vi "calibrate trap data V3RG.vi"(0 "array of calibration clusters":T4(array[cluster]) {"offset_y (mV)" format="%#_2g"; "kappa_y (pN/nm)" min=0.0 step=0.001 format="%#_2g"; "alpha_y (nm/V)" step=10.0 format="%#_3g"; "kappa_x (pN/nm)" min=0.0 step=0.001 format="%#_2g"; "offset_x (mV)" format="%#_2g"; "alpha_x (nm/V)" step=10.0 format="%#_3g"}, 3 "Trap position array":dbl[](array[numeric]), 4 "MCL offset scanning range (V)":T2={"Min X"=5.0, "Max X"=10.0, "Min Y"=5.0, "Max Y"=10.0, "Scan increment"=5.0}, 5 "Multi-MCL offset array":T1(array[cluster]), 6 "two trap offset values":T3={"Trap 1X offset"=array[501 elements], "Trap 2X offset"=array[501 elements]}, 7 "Dynamic offset update":bool, 8 "Multiple-MCL offset?":bool, 9 "x (true) or y (false)":bool, 10 "Data array":waveform(dbl)[](array[waveform]), 11 "Offset File step size":dbl) -> (1 "Positions out":dbl[][](array[numeric]), 2 "Forces out (pN)":dbl[][](array[numeric]))   [LabVIEW 2014]
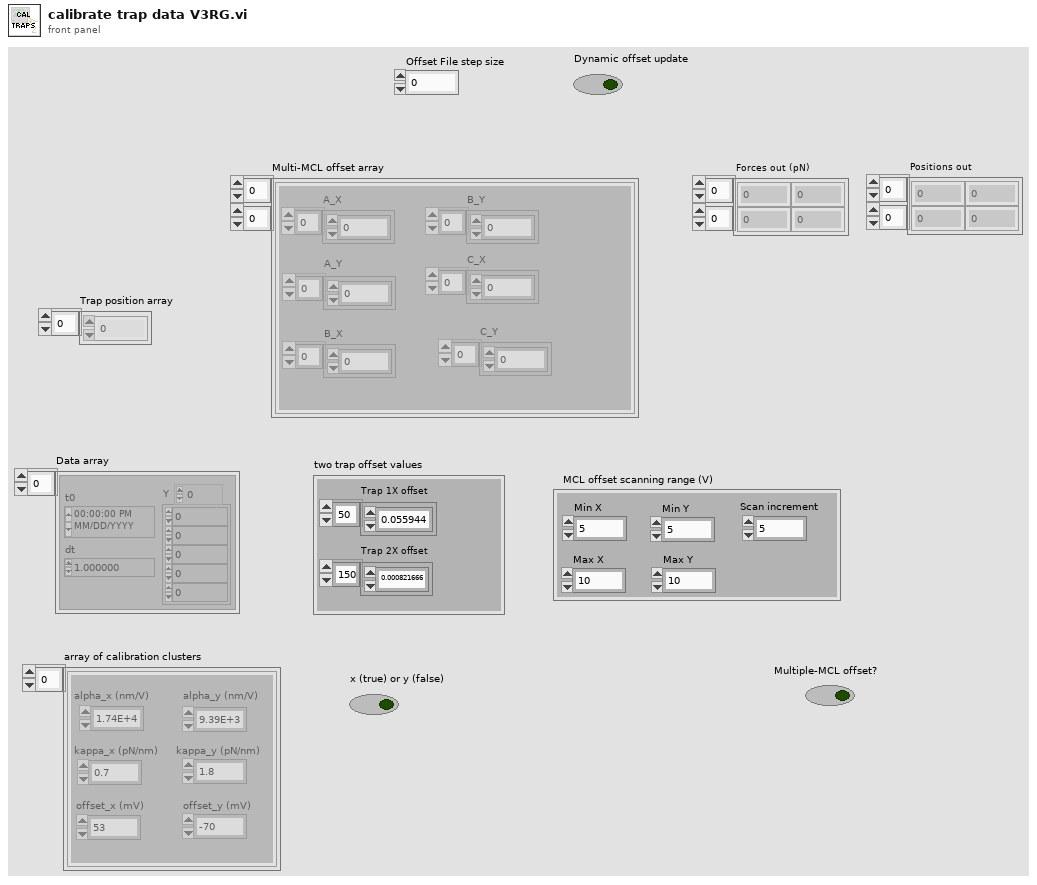
[diagram p1: front panel]
types:
  T1 = cluster{"A_X":dbl[], "A_Y":dbl[], "B_X":dbl[], "B_Y":dbl[], "C_X":dbl[], "C_Y":dbl[]}[][]
  T2 = cluster{"Min X":dbl, "Max X":dbl, "Min Y":dbl, "Max Y":dbl, "Scan increment":dbl}
  T3 = cluster{"Trap 1X offset":dbl[], "Trap 2X offset":dbl[]}
  T4 = cluster{"alpha_x (nm/V)":dbl, "offset_x (mV)":dbl, "kappa_x (pN/nm)":dbl, "alpha_y (nm/V)":dbl, "kappa_y (pN/nm)":dbl, "offset_y (mV)":dbl}[]
  T5 = cluster{"alpha_x (nm/V)":dbl, "offset_x (mV)":dbl, "kappa_x (pN/nm)":dbl, "alpha_y (nm/V)":dbl, "kappa_y (pN/nm)":dbl, "offset_y (mV)":dbl}
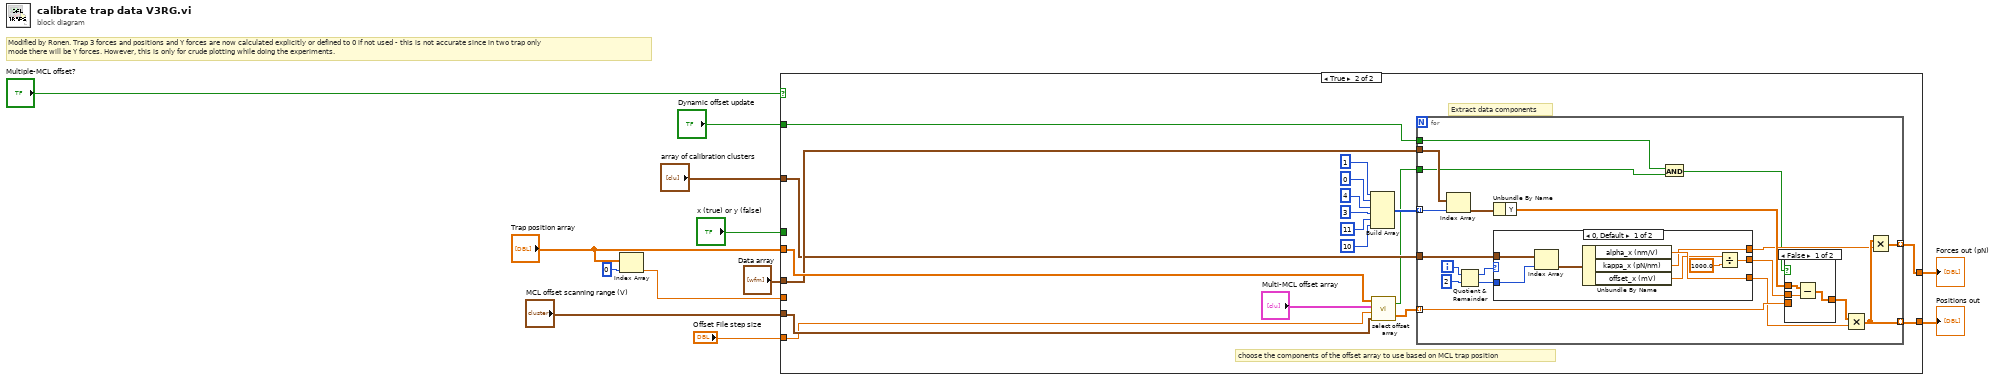
[diagram p0: block diagram]
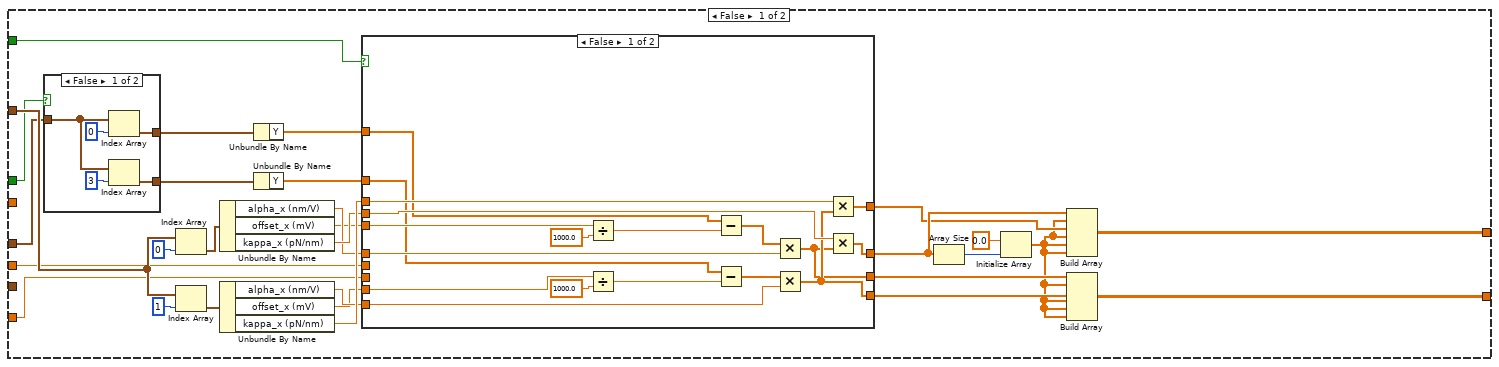
[diagram p2: hidden frame]
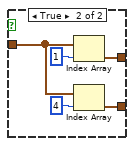
[diagram p3: hidden frame]
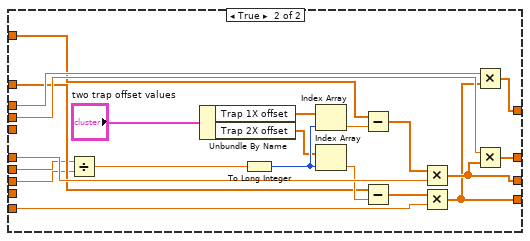
[diagram p4: hidden frame]
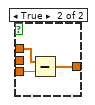
[diagram p5: hidden frame]
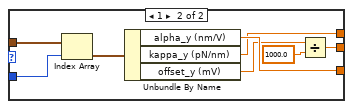
[diagram p6: hidden frame]
diagram:
  # "Modified by Ronen. Trap 3 forces and positions and Y forces are now calculated explicitly or defined to 0 if not used - this is not accurate since in two trap only\nmode there will be Y forces. However, this is only for crude plotting while doing the experiments."
  n1 = Index Array(array="Trap position array", index=0) -> (element=w7:dbl)
  n2 = case shown="True" "Multiple-MCL offset?" {
    tunnel: "Dynamic offset update" -> [w35 w94]
    tunnel: "array of calibration clusters" -> [w34 w95]
    tunnel: "Data array" -> [w29 w98]
    tunnel: w7 -> [w20 _]
    tunnel: "MCL offset scanning range (V)" -> [_ w107]
    tunnel: "Trap position array" -> [_ w108]
    tunnel: "Offset File step size" -> [w19 w97]
    tunnel: [w18 w92] -> w3
    tunnel: [w17 w93] -> w2
    tunnel: "x (true) or y (false)" -> [w16 _]
    frame False {
      n3 = case shown="False" w16 {
        tunnel: w29 -> [w43 w51]
        tunnel: [w44 w48] -> w28
        tunnel: [w42 w47] -> w27
        frame False {
          n4 = Index Array(array=w43, index=0) -> (element=w44:waveform(dbl))
          n5 = Index Array(array=w43, index=3) -> (element=w42:waveform(dbl))
        }
        frame True {
          n6 = Index Array(array=w51, index=1) -> (element=w48:waveform(dbl))
          n7 = Index Array(array=w51, index=4) -> (element=w47:waveform(dbl))
        }
      }
      n8 = Index Array(array=w34, index=0) -> (element=w31:T5)
      n9 = Index Array(array=w34, index=1) -> (element=w30:T5)
      n10 = Unbundle By Name(w31) -> ("alpha_x (nm/V)"=w38:dbl, "offset_x (mV)"=w36:dbl, "kappa_x (pN/nm)"=w40:dbl)
      n11 = Unbundle By Name(w30) -> ("alpha_x (nm/V)"=w39:dbl, "offset_x (mV)"=w37:dbl, "kappa_x (pN/nm)"=w41:dbl)
      n12 = Unbundle By Name(w28) -> ("Y"=w26:dbl[])
      n13 = Unbundle By Name(w27) -> ("Y"=w25:dbl[])
      n14 = case shown="False" w35 {
        tunnel: w36 -> [w63 _]
        tunnel: w37 -> [w62 _]
        tunnel: w38 -> [w61 w83]
        tunnel: w39 -> [w60 w80]
        tunnel: w40 -> [w59 w82]
        tunnel: w41 -> [w58 w79]
        tunnel: w25 -> [w57 w78]
        tunnel: w26 -> [w56 w77]
        tunnel: [w55 w73] -> w14
        tunnel: [w54 w74] -> w15
        tunnel: [w53 w75] -> w21
        tunnel: [w52 w76] -> w22
        tunnel: w20 -> [_ w71]
        tunnel: w19 -> [_ w70]
        frame False {
          n15 = Divide(x=w63, y=1000.0) -> (x/y=w67:dbl)
          n16 = Divide(x=w62, y=1000.0) -> (x/y=w66:dbl)
          n17 = Subtract(x=w56, y=w67) -> (x-y=w65:dbl[])
          n18 = Subtract(x=w57, y=w66) -> (x-y=w64:dbl[])
          n19 = Multiply(x=w65, y=w61) -> (x*y=w53:dbl[])
          n20 = Multiply(x=w64, y=w60) -> (x*y=w55:dbl[])
          n21 = Multiply(x=w58, y=w55) -> (x*y=w54:dbl[])
          n22 = Multiply(x=w59, y=w53) -> (x*y=w52:dbl[])
        }
        frame True {
          n23 = Divide(x=w71, y=w70) -> (x/y=w88:dbl)
          n24 = Unbundle By Name("two trap offset values") -> ("Trap 1X offset"=w85:dbl[], "Trap 2X offset"=w86:dbl[])
          n25 = To Long Integer(number=w88) -> (32bit integer=w87:i32)
          n26 = Index Array(array=w85, index=w87) -> (element=w84:dbl)
          n27 = Index Array(array=w86, index=w87) -> (element=w81:dbl)
          n28 = Subtract(x=w77, y=w84) -> (x-y=w90:dbl[])
          n29 = Subtract(x=w78, y=w81) -> (x-y=w89:dbl[])
          n30 = Multiply(x=w90, y=w83) -> (x*y=w75:dbl[])
          n31 = Multiply(x=w89, y=w80) -> (x*y=w73:dbl[])
          n32 = Multiply(x=w79, y=w73) -> (x*y=w74:dbl[])
          n33 = Multiply(x=w82, y=w75) -> (x*y=w76:dbl[])
        }
      }
      n34 = Array Size(array=w22) -> (size(s)=w24:i32)
      n35 = Initialize Array(0.0, w24) -> (w13:dbl[])
      n36 = Build Array(w22, w13, w15, w13, w13, w13) -> (w18:dbl[][])
      n37 = Build Array(w21, w13, w14, w13, w13, w13) -> (w17:dbl[][])
    }
    frame True {
      # "Extract data components"
      # "choose the components of the offset array to use based on MCL trap position"
      n38 = Build Array(1, 0, 4, 3, 11, 10) -> (w99:i32[])
      n39 = call "select offset array.vi"("MCL offset scanning range (V)"=w107, "Offset File step size"=w97, "Multi-MCL offset array"="Multi-MCL offset array", "Trap position array"=w108) -> ("Out offsets"=w96:dbl[], "In range?"=w91:bool)
      n40 = for {
        tunnel: w99 -> [w127] mode=indexing
        tunnel: w98 -> [w126]
        tunnel: w96 -> [w118] mode=indexing
        tunnel: w95 -> [w120]
        tunnel: w94 -> [w111]
        tunnel: [w114] -> w93 mode=indexing
        tunnel: [w112] -> w92 mode=indexing
        tunnel: w91 -> [w109]
        i -> [w123]
        n41 = Index Array(array=w126, index=w127) -> (element=w125:waveform(dbl))
        n42 = Quotient & Remainder(x=w123, y=2) -> (x-y*floor(x/y)=w122:i32, floor(x/y)=w121:i32)
        n43 = Unbundle By Name(w125) -> ("Y"=w119:dbl[])
        n44 = case shown="0, Default" w122 {
          tunnel: w121 -> [w141 w148]
          tunnel: w120 -> [w140 w149]
          tunnel: [w134 w142] -> w117
          tunnel: [w138 w146] -> w115
          tunnel: [w137 w145] -> w113
          frame 0, Default {
            n45 = Index Array(array=w140, index=w141) -> (element=w139:T5)
            n46 = Unbundle By Name(w139) -> ("alpha_x (nm/V)"=w138:dbl, "kappa_x (pN/nm)"=w137:dbl, "offset_x (mV)"=w136:dbl)
            n47 = Divide(x=w136, y=1000.0) -> (x/y=w134:dbl)
          }
          frame 1 {
            n48 = Index Array(array=w149, index=w148) -> (element=w147:T5)
            n49 = Unbundle By Name(w147) -> ("alpha_y (nm/V)"=w146:dbl, "kappa_y (pN/nm)"=w145:dbl, "offset_y (mV)"=w144:dbl)
            n50 = Divide(x=w144, y=1000.0) -> (x/y=w142:dbl)
          }
        }
        n51 = And(x=w111, y=w109) -> (x .and. y?=w110:bool)
        n52 = case shown="False" w110 {
          tunnel: w119 -> [w130 w133]
          tunnel: w118 -> [_ w132]
          tunnel: w117 -> [w129 _]
          tunnel: [w128 w131] -> w116
          frame False {
            n53 = Subtract(x=w130, y=w129) -> (x-y=w128:dbl[])
          }
          frame True {
            n54 = Subtract(x=w133, y=w132) -> (x-y=w131:dbl[])
          }
        }
        n55 = Multiply(x=w116, y=w115) -> (x*y=w114:dbl[])
        n56 = Multiply(x=w114, y=w113) -> (x*y=w112:dbl[])
      }
    }
  }
  "Forces out (pN)" <- w3
  "Positions out" <- w2
